vi "Write NCh 1Samp (String).vi"(4 "timestamp":timestamp, 6 "index_channel":u32, 8 "error in":errorcluster, 9 "data":string[](array[numeric]), 10 "channels":u32[](array[numeric]), 11 "Writer":refnum<class "Synnax Writer.lvclass">) -> (0 "error out":errorcluster, 3 "Writer Out":refnum<class "Synnax Writer.lvclass">)   [LabVIEW 2026, in "synnax_lib.lvlib" / "Synnax Writer.lvclass"]
uses:
  Synnax Writer.lvclass
  Synnax Writer.lvclass/Synnax Writer.ctl
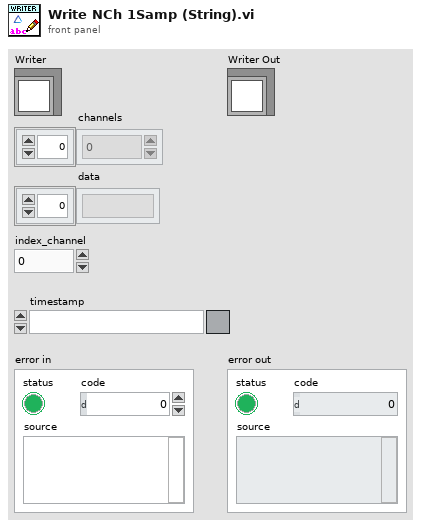
[diagram p1: front panel]
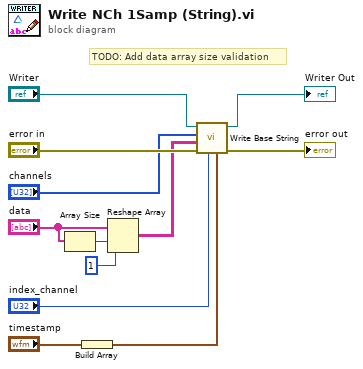
[diagram p0: block diagram]
diagram:
  # "TODO: Add data array size validation"
  n1 = Array Size(array="data") -> (size(s)=w6:i32)
  n2 = Build Array("timestamp") -> (w1:timestamp[])
  n3 = Reshape Array("data", w6, 1) -> (w8:string[][])
  n4 = call "Write Base String.vi"("timestamps"=w1, "index_channel"="index_channel", "error in"="error in", "data"=w8, "channels"="channels", "Writer"="Writer") -> ("error out"=→"error out":errorcluster, "Writer Out"=→"Writer Out":refnum<class "Synnax Writer.lvclass">)  [unwired: 4 in]
